vi "Formula_Node_Ejercicio.vi"() -> ()   [LabVIEW 2020]
panel:
  out "Waveform Graph":dbl[](graph)
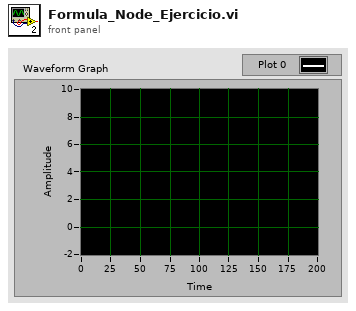
[diagram p1: front panel]
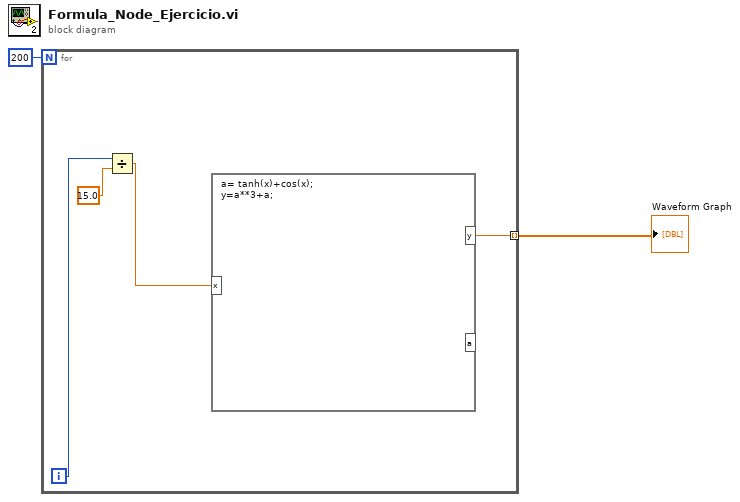
[diagram p0: block diagram]
diagram:
  n1 = for {
    N: 200 -> [_]
    tunnel: [w3] -> w1 mode=indexing
    i -> [w5]
    n2 = Divide(x=w5, y=15.0) -> (x/y=w4:dbl)
    n3 = formula code="a= tanh(x)+cos(x);\ny=a**3+a;"("x"=w4) -> ("y"=w3:dbl)  [unwired: 1 out]
  }
  "Waveform Graph" <- w1
